vi "Update Backlog.vi"(7 "TimingEngine":T1, 8 "error in (no error)":errorcluster, 9 "Backlog":dbl, 11 "FP Controls in":refnum<class "FP Controls.lvclass">) -> (0 "error out":errorcluster, 3 "FP Controls out":refnum<class "FP Controls.lvclass">)   [LabVIEW 2018, in "Configuration Grandmaster.lvlib" / "FP Controls.lvclass"]
uses:
  FP Controls.lvclass
  Common/Controls/TE_Designator.ctl
  FP Controls.lvclass/FP Controls.ctl
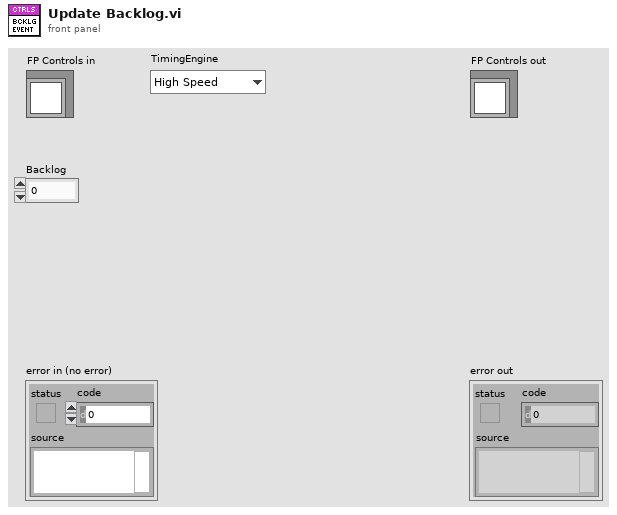
[diagram p1: front panel]
types:
  T1 = typedef "TE_Designator.ctl" = enum16{"High Speed", "Low Speed"}
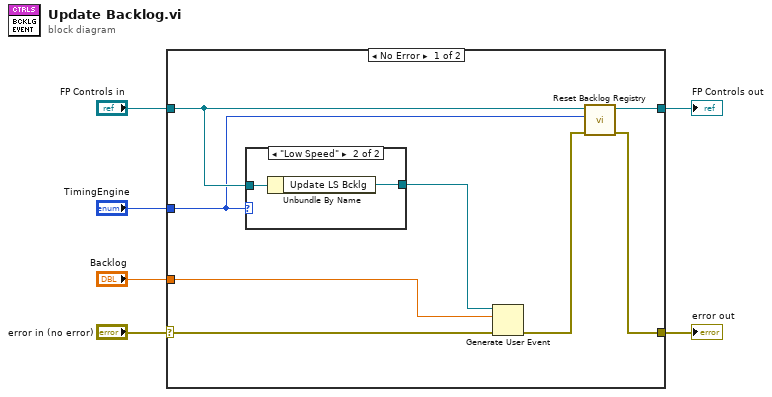
[diagram p0: block diagram]
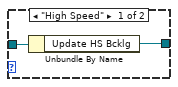
[diagram p2: hidden frame]
diagram:
  n1 = case shown="No Error" "error in (no error)" {
    selector: "error in (no error)" -> [w14 w20]
    tunnel: [w8 w20] -> w5
    tunnel: [w10 w19] -> w3
    tunnel: "FP Controls in" -> [w11 w19]
    tunnel: "Backlog" -> [w12 _]
    tunnel: "TimingEngine" -> [w7 _]
    frame No Error {
      n2 = case shown="\"Low Speed\"" w7 {
        tunnel: w11 -> [w16 w18]
        tunnel: [w15 w17] -> w13
        frame "High Speed" {
          n3 = Unbundle By Name(w16) -> ("Update HS Bcklg"=w15:refnum<user-event>)
        }
        frame "Low Speed" {
          n4 = Unbundle By Name(w18) -> ("Update LS Bcklg"=w17:refnum<user-event>)
        }
      }
      n5 = Generate User Event(user event=w13, event data cluster=w12, error in=w14) -> (error out=w9:errorcluster)  [unwired: 1 in, 1 out]
      n6 = call "Reset Backlog Registry.vi"("error in (no error)"=w9, "TimingEngine"=w7, "FP Controls in"=w11) -> ("error out"=w8:errorcluster, "FP Controls out"=w10:refnum<class "FP Controls.lvclass">)  [unwired: 7 in]
    }
    frame Error {
    }
  }
  "error out" <- w5
  "FP Controls out" <- w3
